vi "Create Lie Group Matrix.vi"(9 "z":dbl, 10 "y":dbl, 11 "x":dbl) -> (2 "real matrix":T1)   [LabVIEW 2017, in "NI_Kinematics.lvlib"]
uses:
  <vilib>/robotics/Kinematics/NI_Kinematics.lvlib
  <vilib>/Analysis/Matrix/Datatypes/RealMatrix.ctl
  <vilib>/Analysis/Matrix/NI_Matrix.lvlib
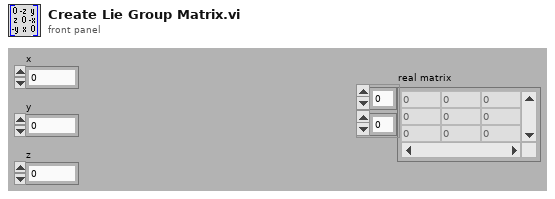
[diagram p1: front panel]
types:
  T1 = typedef "NI_Matrix.lvlib/RealMatrix.ctl" = dbl[][]
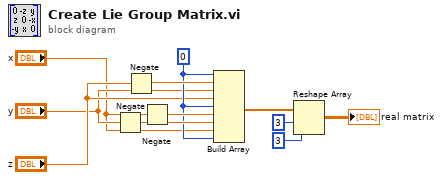
[diagram p0: block diagram]
diagram:
  w5 = 0 ("index")
  n1 = Negate(x="y") -> (-x=w8:dbl)
  n2 = Negate(x="z") -> (-x=w9:dbl)
  n3 = Negate(x="x") -> (-x=w7:dbl)
  n4 = Build Array(w5, w9, "y", "z", w5, w7, w8, "x", w5) -> (w6:dbl[])
  n5 = Reshape Array(w6, 3 ("dimension size"), 3 ("dimension size")) -> (→"real matrix":dbl[][])
